vi "AutoDetector_BiasAdjust.vi"(7 "Auto-Detect Bias info":T3, 11 "ExptParamAndMR":T2) -> (3 "ExptParamAndMR":T2)   [LabVIEW 2015]
uses:
  Controls/Auto-Detector Bias Info.ctl
  Controls/Auto-Detector Peak Info.ctl
  Type/_Mass Range Parameters.ctl
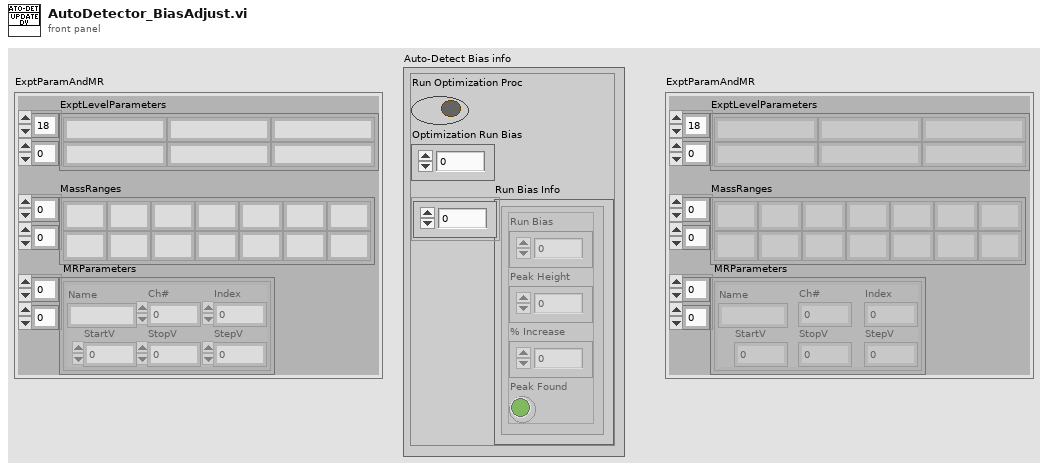
[diagram p1: front panel]
types:
  T1 = typedef "_Mass Range Parameters.ctl" = cluster{"Name":string, "Ch#":u8, "StartV":dbl, "StopV":dbl, "StepV":dbl, "Index":u8}
  T2 = cluster{"ExptLevelParameters":string[][], "MassRanges":string[][], " MRParameters":T1[][]}
  T3 = typedef "Auto-Detector Bias Info.ctl" = cluster{"Run Optimization Proc":bool, "Optimization Run Bias":u32, "Run Bias Info":T4[]}
  T4 = typedef "Auto-Detector Peak Info.ctl" = cluster{"Run Bias":u32, "Peak Height":dbl, "% Increase":dbl, "Peak Found":bool}
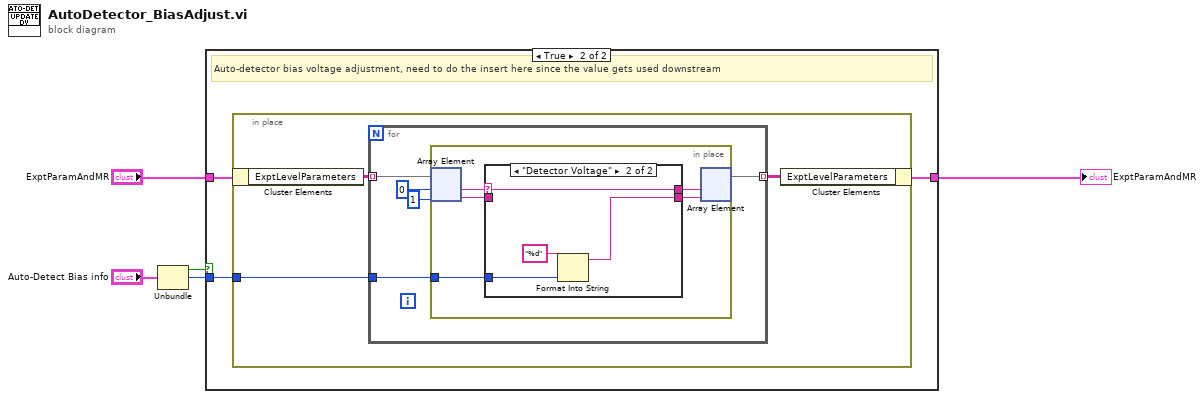
[diagram p0: block diagram]
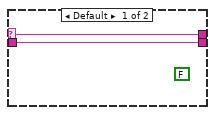
[diagram p3: hidden frame]
diagram:
  n1 = Unbundle("Auto-Detect Bias info") -> ("Run Optimization Proc"=w4:bool, "Optimization Run Bias"=w3:u32)  [unwired: 1 out]
  n2 = case shown="True" w4 {
    tunnel: [w6 w7] -> w1
    tunnel: "ExptParamAndMR" -> [w6 w8]
    tunnel: w3 -> [_ w9]
    frame False {
    }
    frame True {
      # "Auto-detector bias voltage adjustment, need to do the insert here since the value gets used downstream"
      n3 = in-place {
        in-place-border: w9 -> [w12]
        n4 = in-place-cluster #1(w8) -> ("ExptLevelParameters"=w11:string[][])
        n5 = for {
          tunnel: w11 -> [w17] mode=indexing
          tunnel: w12 -> [w16]
          tunnel: [w13] -> w10 mode=indexing
          n6 = in-place {
            in-place-border: w16 -> [w18]
            n7 = in-place-array #2(w17, 0, 1) -> (w22:string, w21:string)
            n8 = case shown="\"Detector Voltage\"" w22 {
              selector: w22 -> [w24 w28]
              tunnel: w21 -> [w23 _]
              tunnel: [w24 w28] -> w20
              tunnel: [w23 w25] -> w19
              tunnel: w18 -> [_ w26]
              frame Default {
                (unwired) FALSE
              }
              frame "Detector Voltage" {
                n9 = Format Into String(format string="%d", w26) -> (resulting string=w25:string)  [unwired: 2 in, 1 out]
              }
            }
            n10 = in-place-array #2(w20, w19) -> (w13:string[])  [unwired: 2 out]
          }
        }
        n11 = in-place-cluster #1("ExptLevelParameters"=w10) -> (w7:T2)
      }
    }
  }
  "ExptParamAndMR" <- w1
